vi "AD5933_SetStatus (NI-845x I2C)(SubVI).vi"(7 "error in":errorcluster, 8 "ConfigRegister (0x80)":u8, 9 "ControlRegisterStates(D15-D12)":T1=2 items=["Initialize with start frequency"=1, "Start frequency sweep"=2, "Increment frequency"=3, "Repeat frequency"=4, "Measure temperature"=9, "Power-down mode"=10, "Standby mode"=11], 10 "NI-845x Config for I2C (in)":cluster{"i2c configuration":T2, "Refnum in":T3}) -> (0 "error out":errorcluster, 3 "NI-845x Config for I2C (out)":T4)   [LabVIEW 2017]
doc: "Set Status of AD933 with NI-845X device."
uses:
  <vilib>/ni845x/ni845x.llb/ni845xI2cConfiguration.ctl
  <vilib>/ni845x/ni845x.llb/ni845xControl.ctl
  TypeDefs/AD5933_OperationState.ctl
  TypeDefs/AD5933_Registers.ctl
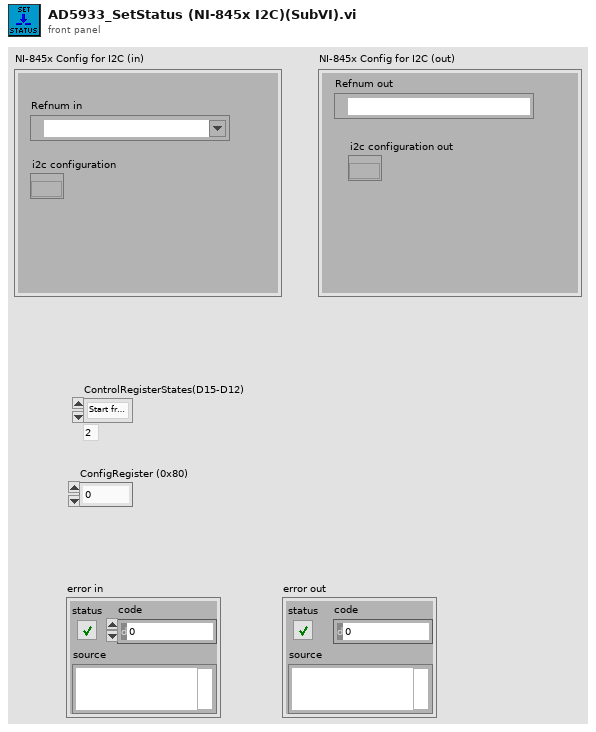
[diagram p1: front panel]
types:
  T1 = typedef "AD5933_OperationState.ctl" = u8
  T2 = typedef "ni845xI2cConfiguration.ctl" = refnum<k20>
  T3 = typedef "ni845xControl.ctl" = refnum<k21>
  T4 = cluster{"i2c configuration out":T2, "Refnum out":T3}
  T5 = typedef "AD5933_Registers.ctl" = u8
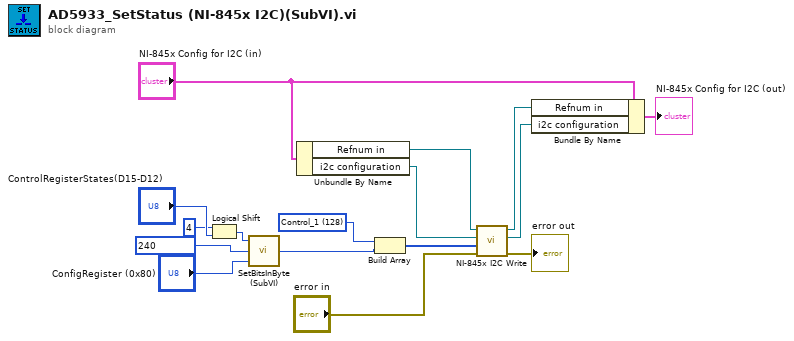
[diagram p0: block diagram]
diagram:
  w1 = T5 128 items=["Control_1"=128, "Control_0"=129, "StartFeq_2"=130, "StartFeq_1"=131, "StartFeq_0"=132, "FreqInc_2"=133, "FreqInc_1"=134, "FreqInc_0"=135, "NumOfInc_1"=136, "NumOfInc_0"=137, "NumOfSetCycl_1"=138, "NumOfSetCycl_0"=139, "Status"=143, "TempData_1"=146, "TempData_0"=147, "RealData_1"=148, "RealData_0"=149, "ImagData_1"=150, "ImagData_0"=151] ("Register")
  n1 = Logical Shift(y=i16 4, x="ControlRegisterStates(D15-D12)") -> (x << y=w5:T1)
  n2 = call "SetBitsInByte (SubVI).vi"("Iput Byte"="ConfigRegister (0x80)", "Bitsmask"=u8 240, "Bits to set"=w5) -> ("Output Byte"=w3:u8)
  n3 = Unbundle By Name("NI-845x Config for I2C (in)") -> ("Refnum in"=w13:T3, "i2c configuration"=w12:T2)
  n4 = Build Array(w1, w3) -> (w2:T5[])
  n5 = call <vilib>:"NI-845x I2C Write.vi"("error in (no error)"="error in", "write data"=w2, "i2c configuration in"=w12, "device reference in"=w13) -> ("error out"=→"error out":errorcluster, "i2c configuration out"=w15:T2, "device reference out"=w14:T3)  [unwired: 5 in]
  n6 = Bundle By Name(cluster="NI-845x Config for I2C (in)", "Refnum in"=w14, "i2c configuration"=w15) -> (→"NI-845x Config for I2C (out)":cluster{"i2c configuration":T2, "Refnum in":T3})
